vi "Set Timing Source.vi"(8 "error in (no error)":errorcluster, 10 "Timing Source":enum16{"Automatic", "Custom Device"}(ring), 11 "Item Ref in":T1 format="%.0x") -> (0 "error out":errorcluster, 3 "Item Ref out":T1 format="%.0x")   [LabVIEW 2020, in "SEECD System Explorer.lvlib"]
uses:
  SEECD System Explorer.lvlib
  C:/Users/Administrator/Desktop/Jatin/All DNC DLLs/NationalInstruments.VeriStand.SystemDefinitionAPI.dll
  Jatin/All DNC DLLs/NationalInstruments.VeriStand.SystemDefinitionAPI.dll
  C:/Users/Administrator/Desktop/Jatin/All DNC DLLs/NationalInstruments.VeriStand.SystemStorage.dll
  Jatin/All DNC DLLs/NationalInstruments.VeriStand.SystemStorage.dll
  <vilib>/NI VeriStand/Custom Device Tools/Custom Device Utility Library/Custom Device Utility Library.lvlib
  <vilib>/NI VeriStand/Custom Device API/Custom Device API.lvlib
  <vilib>/NI VeriStand/Custom Device API/Custom Device Item Ref.ctl
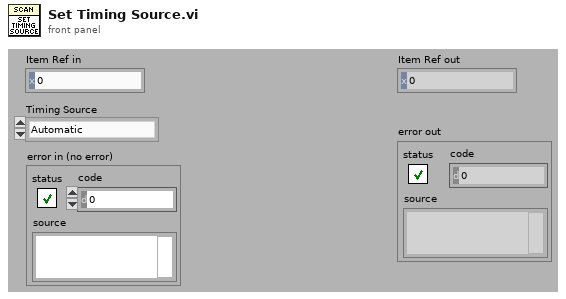
[diagram p1: front panel]
types:
  T1 = typedef "Custom Device API.lvlib/Custom Device Item Ref.ctl" = u64
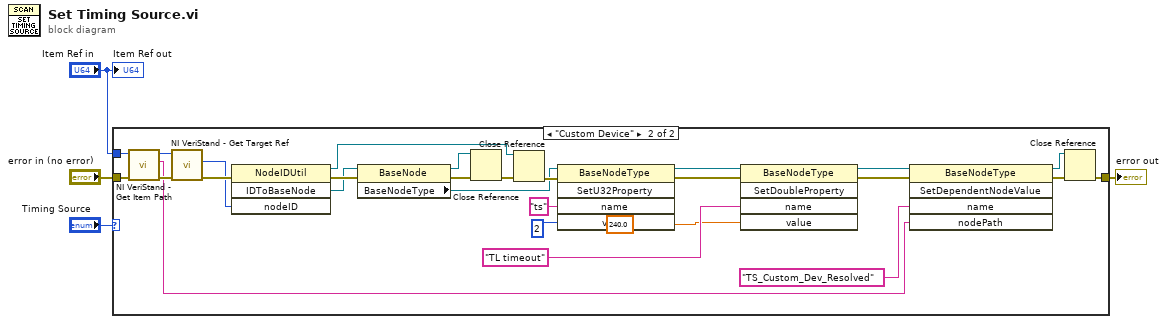
[diagram p0: block diagram]
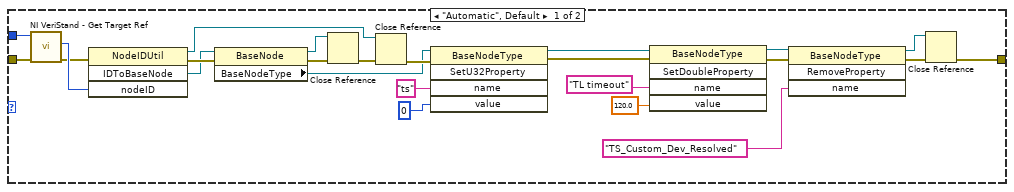
[diagram p2: hidden frame]
diagram:
  n1 = case shown="\"Custom Device\"" "Timing Source" {
    tunnel: "Item Ref in" -> [w27 w55]
    tunnel: "error in (no error)" -> [w28 w54]
    tunnel: [w21 w45] -> w2
    frame "Automatic", Default {
      n2 = call <vilib>:"NI VeriStand - Get Target Ref.vi"("error in"=w28, "Item Ref in"=w27) -> ("error out"=w5:errorcluster, "Target Ref"=w6:T1)  [unwired: 6 in, 2 out]
      n3 = invoke class="NodeIDUtil" method="IDToBaseNode"(error in=w5, "nodeID"=w6) -> (reference out=w11:refnum<k39>, error out=w10:errorcluster, "IDToBaseNode"=w9:refnum<k39>)  [unwired: 2 in, 1 out]
      n4 = property class="BaseNode"(reference=w9, error in=w10) -> (reference out=w13:refnum<k39>, error out=w12:errorcluster, "BaseNodeType"=w7:refnum<k39>)
      n5 = Close Reference(reference=w13, error in (no error)=w12) -> (error out=w14:errorcluster)
      n6 = Close Reference(reference=w11, error in (no error)=w14) -> (error out=w8:errorcluster)
      n7 = invoke class="BaseNodeType" method="SetU32Property"(reference=w7, error in=w8, "name"="ts", "value"=u32 0) -> (reference out=w19:refnum<k39>, error out=w16:errorcluster)  [unwired: 1 in, 3 out]
      n8 = invoke class="BaseNodeType" method="SetDoubleProperty"(reference=w19, error in=w16, "name"="TL timeout", "value"=120.0) -> (reference out=w18:refnum<k39>, error out=w17:errorcluster)  [unwired: 1 in, 3 out]
      n9 = invoke class="BaseNodeType" method="RemoveProperty"(reference=w18, error in=w17, "name"="TS_Custom_Dev_Resolved") -> (reference out=w23:refnum<k39>, error out=w22:errorcluster)  [unwired: 1 in, 2 out]
      n10 = Close Reference(reference=w23, error in (no error)=w22) -> (error out=w21:errorcluster)
    }
    frame "Custom Device" {
      n11 = call <vilib>:"NI VeriStand - Get Item Path.vi"("error in (no error)"=w54, "Item Ref in"=w55) -> ("error out"=w53:errorcluster, "Path"=w49:string, "Item Ref out"=w52:T1)  [unwired: 6 in, 1 out]
      n12 = call <vilib>:"NI VeriStand - Get Target Ref.vi"("error in"=w53, "Item Ref in"=w52) -> ("error out"=w32:errorcluster, "Target Ref"=w29:T1)  [unwired: 6 in, 2 out]
      n13 = invoke class="NodeIDUtil" method="IDToBaseNode"(error in=w32, "nodeID"=w29) -> (reference out=w35:refnum<k39>, error out=w34:errorcluster, "IDToBaseNode"=w33:refnum<k39>)  [unwired: 2 in, 1 out]
      n14 = property class="BaseNode"(reference=w33, error in=w34) -> (reference out=w37:refnum<k39>, error out=w36:errorcluster, "BaseNodeType"=w30:refnum<k39>)
      n15 = Close Reference(reference=w37, error in (no error)=w36) -> (error out=w38:errorcluster)
      n16 = Close Reference(reference=w35, error in (no error)=w38) -> (error out=w31:errorcluster)
      n17 = invoke class="BaseNodeType" method="SetU32Property"(reference=w30, error in=w31, "name"="ts", "value"=u32 2) -> (reference out=w43:refnum<k39>, error out=w44:errorcluster)  [unwired: 1 in, 3 out]
      n18 = invoke class="BaseNodeType" method="SetDoubleProperty"(reference=w43, error in=w44, "name"="TL timeout", "value"=240.0) -> (reference out=w42:refnum<k39>, error out=w41:errorcluster)  [unwired: 1 in, 3 out]
      n19 = invoke class="BaseNodeType" method="SetDependentNodeValue"(reference=w42, error in=w41, "name"="TS_Custom_Dev_Resolved", "nodePath"=w49) -> (reference out=w47:refnum<k39>, error out=w46:errorcluster)  [unwired: 1 in, 3 out]
      n20 = Close Reference(reference=w47, error in (no error)=w46) -> (error out=w45:errorcluster)
    }
  }
  "error out" <- w2
  "Item Ref out" <- "Item Ref in"
